vi "Read ref.vi"(8 "error in (no error)":errorcluster, 11 "DapperRow in":refnum<class "DapperRow.lvclass">) -> (0 "error out":errorcluster, 2 "ref":refnum<k24>, 3 "DapperRow out":refnum<class "DapperRow.lvclass">)   [LabVIEW 2020, in "ORM_Dapper.lvlib" / "DapperRow.lvclass"]
uses:
  DapperRow.lvclass
  DapperRow.lvclass/DapperRow.ctl
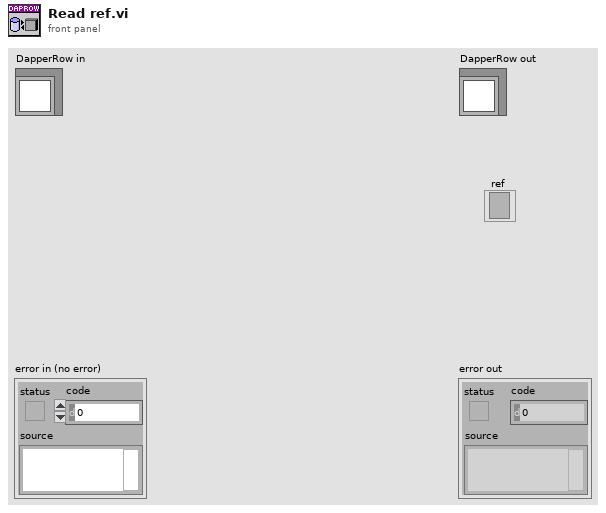
[diagram p1: front panel]
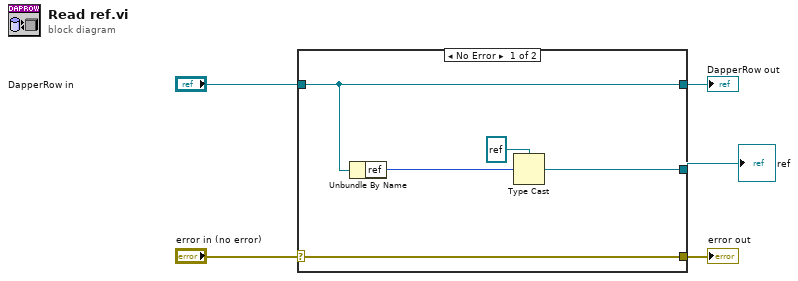
[diagram p0: block diagram]
diagram:
  n1 = case shown="No Error" "error in (no error)" {
    selector: "error in (no error)" -> [w10 w11]
    tunnel: [w10 w11] -> w4
    tunnel: [w9 w12] -> w2
    tunnel: "DapperRow in" -> [w9 w12]
    tunnel: [w7 _] -> w1
    frame No Error {
      n2 = Unbundle By Name(w9) -> ("ref"=w8:u64)
      n3 = Type Cast(type=refnum<k24> refnum ("ref"), x=w8) -> (*(type *) &x=w7:refnum<k24>)
    }
    frame Error {
    }
  }
  "error out" <- w4
  "DapperRow out" <- w2
  "ref" <- w1
